vi "Test - Get JSON Type from LV Type.vi"   [LabVIEW 2020, in "JSON Schema Generator.lvlib"]
uses:
  JSON Schema Generator.lvlib
  <vilib>/addons/_JKI Toolkits/Caraya/classes/Test/Test.lvclass
  0547ed6d-57df-46aa-a813-f64a6d4eb2f4.vi
  <vilib>/Utility/Data Type/Type Definitions/Data Type.ctl
  <vilib>/Utility/Data Type/NI_Data Type.lvlib
  <vilib>/addons/_JKI Toolkits/Caraya/classes/Assert/Assert.lvclass
  <vilib>/addons/_JKI Toolkits/Caraya/classes/Assert/Assert Equal Value_Variant.vi
  <vilib>/addons/_JKI Toolkits/Caraya/classes/Assert/Assert Error.vi
types:
  T1 = typedef "NI_Data Type.lvlib/Data Type.ctl" = enum8{"Invalid Type", "Void", "I8", "I16", "I32", "I64", "U8", "U16", "U32", "U64", "Single Float", "Double Float", "Extended Float", "Single Complex", "Double Complex", "Extended Complex", "Enum U8", "Enum U16", "Enum U32", "Enum U64", "Single Float With Unit", "Double Float With Unit", "Extended Float With Unit", "Single Complex with Unit", "Double Complex with Unit", "Extended Complex with Unit", "Boolean", "String", "Path", "Picture", "Tag", "Array", "Cluster", "Variant", "LV Variant", "Waveform", "Timestamp", "Digital Waveform", "Digital Data", "ExpressData", "Refnum", "External Data", "VI", "Poly VI", "LabVIEW Class Instance", "Fixed Point", "Set Collection", "Map Collection"}
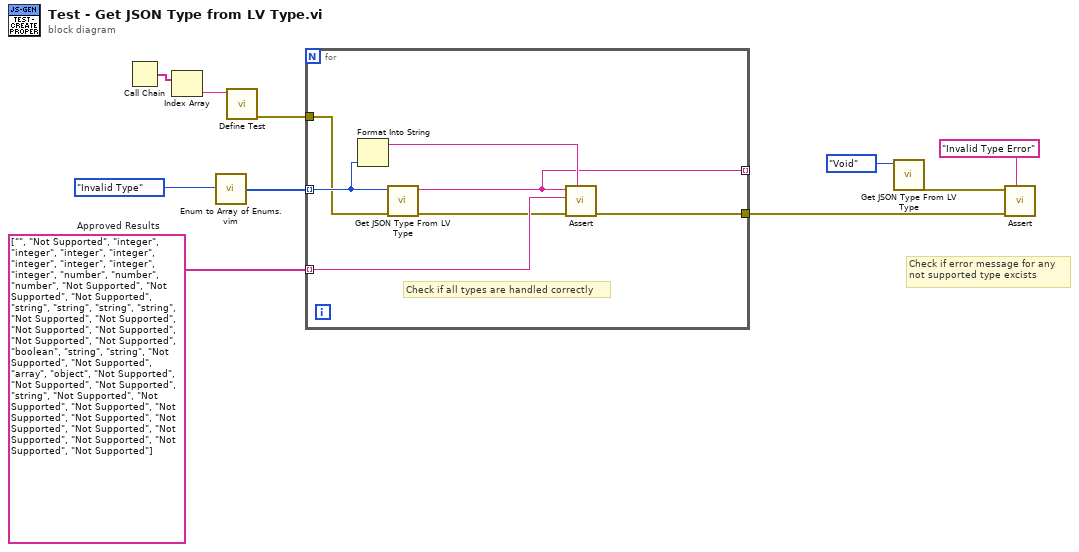
[diagram p0: block diagram]
diagram:
  w5 = string[] ["", "Not Supported", "integer", "integer", "integer", "integer", "integer", "integer", "integer", "integer", "number", "number", "number", "Not Supported", "Not Supported", "Not Supported", "string", "string", "string", "string", "Not Supported", "Not Supported", "Not Supported", "Not Supported", "Not Supported", "Not Supported", "boolean", "string", "string", "Not Supported", "Not Supported", "array", "object", "Not Supported", "Not Supported", "Not Supported", "string", "Not Supported", "Not Supported", "Not Supported", "Not Supported", "Not Supported", "Not Supported", "Not Supported", "Not Supported", "Not Supported", "Not Supported", "Not Supported"]  # Approved Results
  # "Check if error message for any\nnot supported type excists"
  n1 = Call Chain() -> (call chain=w10:string[])
  n2 = Index Array(array=w10) -> (element=w9:string)  [unwired: 1 in]
  n3 = call "Enum to Array of Enums.vim"("enum"=Data_Type."Invalid Type" ("Labview Datatype")) -> ("array of enums"=w7:T1[])
  n4 = call <vilib>:"Define Test.vi"("Label (VI Title)"=w9) -> ("error out"=w6:errorcluster)  [unwired: 9 in, 1 out]
  n5 = for {
    tunnel: w7 -> [w16] mode=indexing
    tunnel: w5 -> [w15] mode=indexing
    tunnel: w6 -> [w12]
    tunnel: [w13] -> _ mode=indexing
    tunnel: [w11] -> w1
    # "Check if all types are handled correctly"
    n6 = Format Into String(w16) -> (resulting string=w14:string)  [unwired: 3 in, 1 out]
    n7 = call "Get JSON Type From LV Type.vi"("Labview Datatype"=w16) -> ("JSON Schema Type"=w13:string)  [unwired: 9 in, 1 out]
    n8 = call-poly <vilib>:"Assert.vi"("Label"=w14, "error in (no error)"=w12, "Actual"=w15, "Expected"=w13) -> ("error out"=w11:errorcluster)  [unwired: 6 in, 1 out]
  }
  n9 = call "Get JSON Type From LV Type.vi"("Labview Datatype"=Data_Type."Void") -> ("error out"=w3:errorcluster)  [unwired: 9 in, 1 out]
  n10 = call-poly <vilib>:"Assert.vi"("Label"="Invalid Type Error", "error in (no error)"=w1, "Error?"=w3) -> ()  [unwired: 7 in, 2 out]
